vi "Initialize UI.vi"(8 "error in (no error)":errorcluster, 11 "QControlWizard in":refnum<class "QControl Creation Wizard.lvclass">) -> (0 "error out":errorcluster, 3 "QControlWizard out":refnum<class "QControl Creation Wizard.lvclass">)   [LabVIEW 2020, in "QControl Creation Wizard.lvclass"]
doc: "<b> </b> <b> </b>\n©2016 Q Software Innovations, LLC (QSI)\nwritten by Quentin Alldredge\nproduced in LabVIEW 2015\n\nsupport@qsoftwareinnovations.com\nwww.qsoftwareinnovations.com\n\nAll rights reserved.\n\nRedistribution and use in source and binary forms, with or without modification, are permitted provided that the following conditions are met:\n\n * Redistributions of source code must retain the above copyright notice, this list of conditions and the following disclaimer.\n * Redistributions in binary form must reproduce the above copyright notice, this list of conditions and the following disclaimer in the documentation and/or other materials provided with the distribution.\n * Neither the name of Q Software Innovations, LLC. nor the names of its contributors may be used to endorse or promote products derived from this software without specific prior written permission.\n\nTHIS SOFTWARE IS PROVIDED BY THE COPYRIGHT HOLDERS AND CONTRIBUTORS \"AS IS\" AND ANY EXPRESS OR IMPLIED WARRANTIES, INCLUDING, BUT NOT LIMITED TO, THE IMPLIED WARRANTIES OF MERCHANTABILITY AND FITNESS FOR A PARTICULAR PURPOSE ARE DISCLAIMED. IN NO EVENT SHALL THE COPYRIGHT OWNER OR CONTRIBUTORS BE LIABLE FOR ANY DIRECT, INDIRECT, INCIDENTAL, SPECIAL, EXEMPLARY, OR CONSEQUENTIAL DAMAGES (INCLUDING, BUT NOT LIMITED TO, PROCUREMENT OF SUBSTITUTE GOODS OR SERVICES; LOSS OF USE, DATA, OR PROFITS; OR BUSINESS INTERRUPTION) HOWEVER CAUSED AND ON ANY THEORY OF LIABILITY, WHETHER IN CONTRACT, STRICT LIABILITY, OR TORT (INCLUDING NEGLIGENCE OR OTHERWISE) ARISING IN ANY WAY OUT OF THE USE OF THIS SOFTWARE, EVEN IF ADVISED OF THE POSSIBILITY OF SUCH DAMAGE."
uses:
  QControl Creation Wizard.lvclass
  QControl Creation Wizard.lvclass/QControl Creation Wizard.ctl
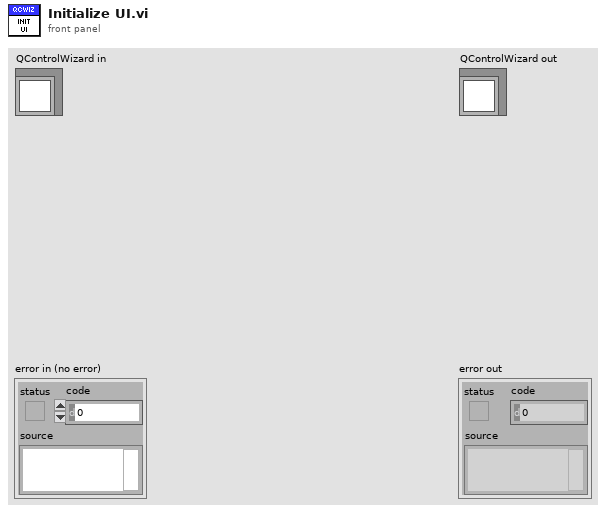
[diagram p1: front panel]
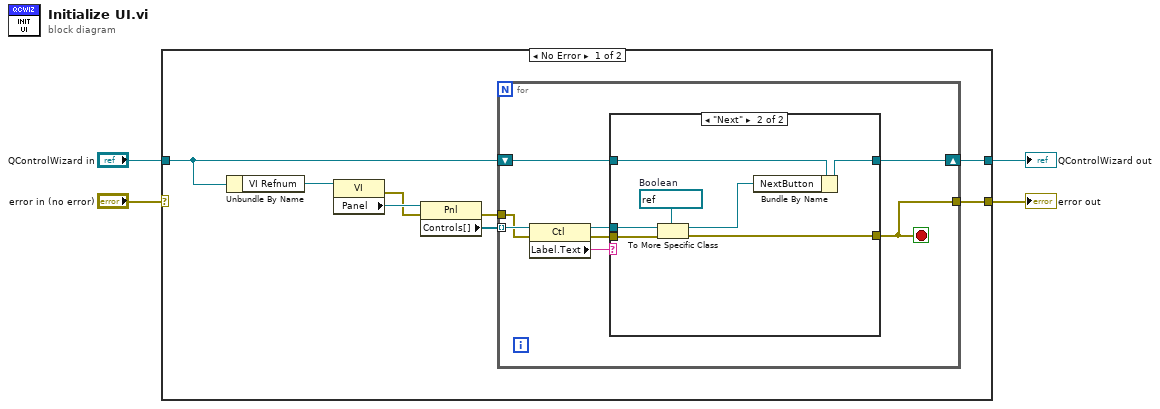
[diagram p0: block diagram]
diagram:
  n1 = case shown="No Error" "error in (no error)" {
    selector: "error in (no error)" -> [_ w30]
    tunnel: [w5 w30] -> w3
    tunnel: [w8 w29] -> w1
    tunnel: "QControlWizard in" -> [w9 w29]
    frame No Error {
      n2 = Unbundle By Name(w9) -> ("VI Refnum"=w12:refnum<vi>)
      n3 = property class="VI"(reference=w12) -> (error out=w7:errorcluster, "Panel"=w11:refnum<vi>)  [unwired: 1 in, 1 out]
      n4 = property class="Pnl"(reference=w11, error in=w7) -> (error out=w6:errorcluster, "Controls[]"=w10:refnum<vi>[])  [unwired: 1 out]
      n5 = for {
        tunnel: w10 -> [w20] mode=indexing
        shift-right: [w16] -> w8
        shift-left: w9 -> [w18]
        tunnel: w6 -> [w15]
        tunnel: [w13] -> w5
        stop <- w13 stop-if-true
        n6 = property class="Ctl"(reference=w20, error in=w15) -> (reference out=w17:refnum<vi>, error out=w14:errorcluster, "Label.Text"=w19:string)
        n7 = case shown="\"Next\"" w19 {
          tunnel: w18 -> [w21 w28]
          tunnel: w17 -> [_ w27]
          tunnel: [w21 w24] -> w16
          tunnel: w14 -> [_ w23]
          tunnel: [_ w22] -> w13
          frame Default {
          }
          frame "Next" {
            w26 = refnum<vi> refnum  # Boolean
            n8 = To More Specific Class(target class=w26, reference=w27, error in=w23) -> (specific class reference=w25:refnum<vi>, error out=w22:errorcluster)
            n9 = Bundle By Name(cluster=w28, "NextButton"=w25) -> (w24:refnum<class "QControl Creation Wizard.lvclass">)
          }
        }
      }
    }
    frame Error {
    }
  }
  "error out" <- w3
  "QControlWizard out" <- w1
